vi "SVFA Wrap or Unwrap Phase (XY) (N Ch).vi"(0 "phase spectra in":cluster{"X":dbl[], "phase":dbl[]}[](array[cluster]) {"phase" format="%.2f"; "X" format="%.2f"}, 1 "desired wrapping":T8(ring)=enum."Wrap: -180 to 180", 2 "custom wrap range":T1={"minimum phase"=-inf, "maximum phase"=inf}, 4 "spectrum info":T2[](array[typedef]) {"x-axis units" items=["Time (s)"=0, "Frequency-CB (Hz)"=1, "Frequency-CPB (Hz)"=1248, "Frequency-Arbitrary (Hz)"=2357, "Quefrency (s)"=2, "Revolutions (rev)"=3, "Order"=4, "Speed (RPM)"=11, "Speed (rad/s)"=21, "Index"=65535]; "weighting filter" items=["Linear", "A-weighting", "B-weighting", "C-weighting", "ITU-R 468-4", "Dolby", "CCITT", "C-message", "Wb", "Wc", "Wd", "We", "Wf", "Wh", "Wj", "Wk", "Wm", "AES17 20 kHz lowpass", "AES17 40 kHz lowpass", "AES17 20 kHz highpass", "AES17 40 kHz highpass"]; "dB reference [EU]" format="%.2f"; "engineering units" items=["custom..."=0, "V"=1, "A"=21, "C"=30, "pC"=31, "s"=32, "-"=29, "Pa"=2, "N"=20, "g"=3, "m/s^2"=4, "m/s"=5, "m"=6, "mm/s"=12, "mm"=13, "micron/s"=14, "micron"=15, "in/s^2"=7, "in/s"=8, "in"=9, "mil/s"=10, "mil"=11, "rad/s^2"=16, "rad/s"=17, "rad"=18, "deg/s^2"=26, "deg/s"=27, "deg"=28, "RPM"=22, "cycle/s^2"=23, "Hz"=24, "cycle"=25, "strain"=19]; "spectral info"."window" items=["None "=0, "Hanning"=1, "Hamming"=2, "Blackman-Harris"=3, "Exact Blackman"=4, "Blackman"=5, "Flat Top"=6, "4 Term B-Harris "=7, "7 Term B-Harris"=8, "Low Sidelobe"=9, "Force - Exponential"=10, "Gaussian"=62]}, 5 "error in (no error)":errorcluster) -> (14 "phase spectra out":cluster{"X":dbl[], "phase":dbl[]}[](array[cluster]) {"phase" format="%.2f"; "X" format="%.2f"}, 15 "unit labels":string[](array[string]), 18 "dup spectrum info":T2[](array[typedef]) {"x-axis units" items=["Time (s)"=0, "Frequency-CB (Hz)"=1, "Frequency-CPB (Hz)"=1248, "Frequency-Arbitrary (Hz)"=2357, "Quefrency (s)"=2, "Revolutions (rev)"=3, "Order"=4, "Speed (RPM)"=11, "Speed (rad/s)"=21, "Index"=65535]; "weighting filter" items=["Linear", "A-weighting", "B-weighting", "C-weighting", "ITU-R 468-4", "Dolby", "CCITT", "C-message", "Wb", "Wc", "Wd", "We", "Wf", "Wh", "Wj", "Wk", "Wm", "AES17 20 kHz lowpass", "AES17 40 kHz lowpass", "AES17 20 kHz highpass", "AES17 40 kHz highpass"]; "dB reference [EU]" format="%.2f"; "engineering units" items=["custom..."=0, "V"=1, "A"=21, "C"=30, "pC"=31, "s"=32, "-"=29, "Pa"=2, "N"=20, "g"=3, "m/s^2"=4, "m/s"=5, "m"=6, "mm/s"=12, "mm"=13, "micron/s"=14, "micron"=15, "in/s^2"=7, "in/s"=8, "in"=9, "mil/s"=10, "mil"=11, "rad/s^2"=16, "rad/s"=17, "rad"=18, "deg/s^2"=26, "deg/s"=27, "deg"=28, "RPM"=22, "cycle/s^2"=23, "Hz"=24, "cycle"=25, "strain"=19]; "spectral info"."window" items=["None "=0, "Hanning"=1, "Hamming"=2, "Blackman-Harris"=3, "Exact Blackman"=4, "Blackman"=5, "Flat Top"=6, "4 Term B-Harris "=7, "7 Term B-Harris"=8, "Low Sidelobe"=9, "Force - Exponential"=10, "Gaussian"=62]}, 19 "error out":errorcluster)   [LabVIEW 2017]
doc: "Wraps the phase spectra to the specified range, so that all phase values are coerced to the specified band. You also can use this VI to unwrap phase spectra to eliminate discontinuities with absolute values exceeding 180 degrees = pi radians = 0.5 cycles. Wire data to the <B>phase spectrum in</B> input to determine the polymorphic instance to use or manually select the instance."
uses:
  <vilib>/addons/_NISVFA/_Shared subVIs/Controls/svc_Spectrum Info.ctl
  <vilib>/addons/_NISVFA/_Shared subVIs/Controls/svc_X-Axis Units.ctl
  <vilib>/addons/_NISVFA/_Shared subVIs/Controls/svc_Spectrum Type.ctl
  <vilib>/addons/_NISVFA/_Shared subVIs/Controls/svc_Engineering Units Text Ring.ctl
  <vilib>/addons/_NISVFA/_Shared subVIs/Controls/svc_Weighting Filter Text Ring.ctl
  <vilib>/addons/_NISVFA/_Shared subVIs/Controls/svc_Complimentary Spectrum Units.ctl
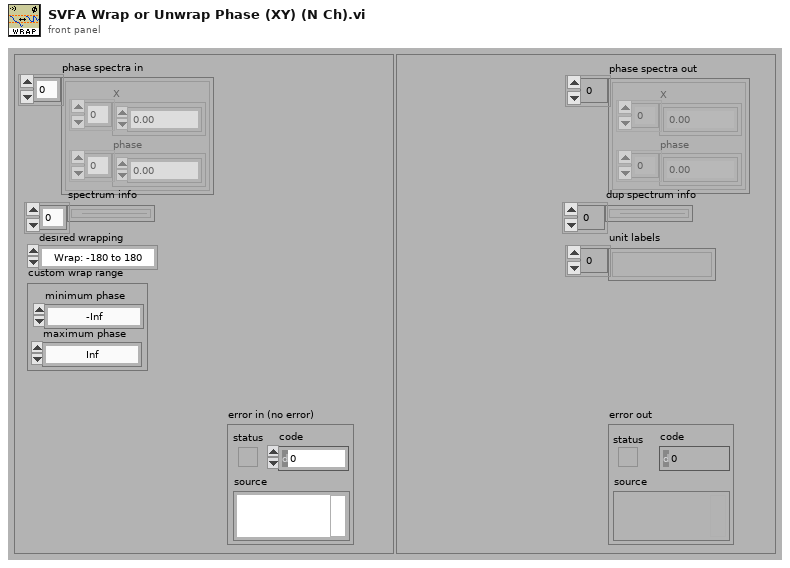
[diagram p1: front panel]
types:
  T1 = cluster{"minimum phase":dbl, "maximum phase":dbl}
  T2 = typedef "svc_Spectrum Info.ctl" = cluster{"channel name":string, "description":string, "x-axis units":T3, "spectral info":cluster{"spectrum type":T4, "linear/dB":enum16{"linear", "dB"}, "window":u16, "window size":i32, "FFT size":i32}, "engineering units":T5, "custom label":string, "dB reference [EU]":dbl, "peak units":enum16{"rms", "peak", "peak-peak"}, "weighting filter":T6, "spectral density?":bool, "unit label":string, "spectrum skewed?":bool, "complimentary spectrum units":T7}
  T3 = typedef "svc_X-Axis Units.ctl" = u16
  T4 = typedef "svc_Spectrum Type.ctl" = enum16{"FFT Spectrum [complex]", "Amplitude [Magnitude]", "Power [Magnitude^2]", "Cross Spectrum [complex]", "Frequency Response [Complex]"}
  T5 = typedef "svc_Engineering Units Text Ring.ctl" = u16
  T6 = typedef "svc_Weighting Filter Text Ring.ctl" = u16
  T7 = typedef "svc_Complimentary Spectrum Units.ctl" = enum16{"none", "radians", "degrees", "cycles", "imaginary"}
  T8 = enum16{"No change", "Unwrap", "Wrap: -360 to 0", "Wrap: -270 to 90", "Wrap: -180 to 180", "Wrap: -90 to 270", "Wrap: 0 to 360", "Wrap: custom range"}
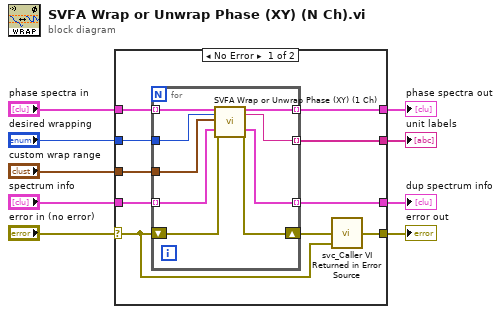
[diagram p0: block diagram]
diagram:
  n1 = case shown="No Error" "error in (no error)" {
    selector: "error in (no error)" -> [w16 w30]
    tunnel: "phase spectra in" -> [w18 w31]
    tunnel: [w17 w31] -> w8
    tunnel: [w19 w30] -> w6
    tunnel: "desired wrapping" -> [w12 _]
    tunnel: "spectrum info" -> [w14 w29]
    tunnel: [w13 w29] -> w3
    tunnel: "custom wrap range" -> [w11 _]
    tunnel: [w10 _] -> w1
    frame No Error {
      n2 = for {
        tunnel: w18 -> [w28] mode=indexing
        tunnel: [w27] -> w17 mode=indexing
        shift-right: [w25] -> w15
        shift-left: w16 -> [w26]
        tunnel: w14 -> [w24] mode=indexing
        tunnel: [w23] -> w13 mode=indexing
        tunnel: w12 -> [w22]
        tunnel: w11 -> [w21]
        tunnel: [w20] -> w10 mode=indexing
        n3 = call <vilib>:"SVFA Wrap or Unwrap Phase (XY) (1 Ch).vi"("phase spectrum in"=w28, "desired wrapping"=w22, "custom wrap range"=w21, "spectrum info"=w24, "error in (no error)"=w26) -> ("phase spectrum out"=w27:cluster{"X":dbl[], "phase":dbl[]}, "unit label"=w20:string, "dup spectrum info"=w23:T2, "error out"=w25:errorcluster)  [unwired: 11 in]
      }
      n4 = call <vilib>:"svc_Caller VI Returned in Error Source.vi"("warning input to caller"=w16, "error in (no error)"=w15) -> ("error out"=w19:errorcluster)  [unwired: 3 in]
    }
    frame Error {
    }
  }
  "phase spectra out" <- w8
  "error out" <- w6
  "dup spectrum info" <- w3
  "unit labels" <- w1
